vi "Cuadrada.vi"() -> ()   [LabVIEW 2017]
panel:
  in  "Cuadrada":bool
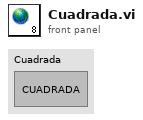
[diagram p1: front panel]
diagram:
